vi "niRFUtil RFHS Channelizer ChannelizerArray CSG  phaseII.vi"(0 "Channelizer Ref":refnum<data-value>, 1 "Reset":bool, 2 "Benchmark Task":T2, 5 "Data":csg[](array[numeric]), 7 "Data Subset":T1={"Offset"=0, "Length"=-1}, 11 "error in (no error)":errorcluster, 13 "CPU Context":string) -> (4 "Channelizer Ref (out)":refnum<data-value>, 6 "Channel Data":csg[](array[numeric]), 8 "Channel Data Len":u32[](array[numeric]), 15 "error out":errorcluster)   [LabVIEW 2015, in "niRFUtil.lvlib"]
uses:
  niRFUtil.lvlib
  Utilities/Benchmark/niRFUtil RFHS Benchmark Task.ctl
  Utilities/niRFUtil RFHS Util Data Subset.ctl
  Includes/niRFUtil RFHS Channelizer ChannelizerInfo CSG.ctl
  Includes/niRFUtil RFHS Channelizer FilterRef.ctl
  Includes/niRFUtil RFHS Channelizer ChannelizerBufferingMode.ctl
  Utilities/Data FIFO/niRFUtil RFHS FIFO Reference.ctl
  Utilities/Data FIFO/niRFUtil RFHS FIFO.ctl
  Includes/niRFUtil RFHS Channelizer ChannelizerType.ctl
  Includes/niRFUtil RFHS Channelizer ChannelizerFlags.ctl
  niRFUtil RFHS Channelizer AdjustDataSubsetSpecification.vi
  niRFUtil RFHS Channelizer BufferLen CSG.vi
  niRFUtil RFHS Channelizer ChannelizerHandleDllError.vi
  Utilities/niRFUtil RFHS Util Process CPU Context.vi
  niRFUtil RFHS Channelizer ProcessCPUContext.vi
  Utilities/niRFUtil RFHS Util Dll Path.vi
panel:
  out "Time":u32
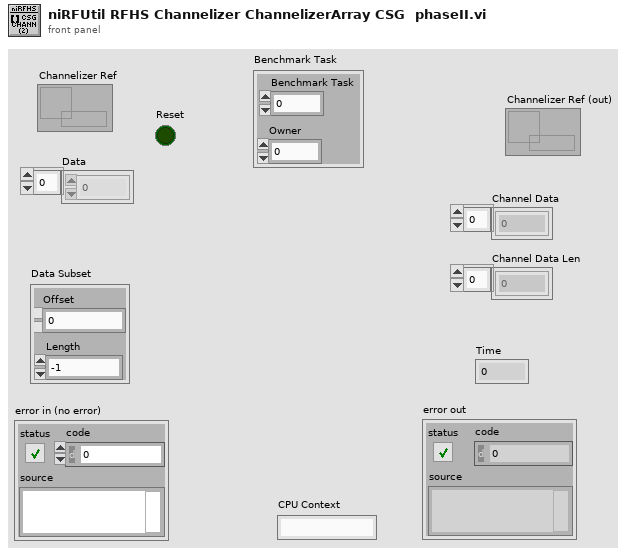
[diagram p1: front panel]
types:
  T1 = typedef "niRFUtil.lvlib/niRFUtil RFHS Util Data Subset.ctl" = cluster{"Offset":i32, "Length":i32}
  T2 = typedef "niRFUtil.lvlib/niRFUtil RFHS Benchmark Task.ctl" = cluster{"Benchmark Task":u64, "Owner":u32}
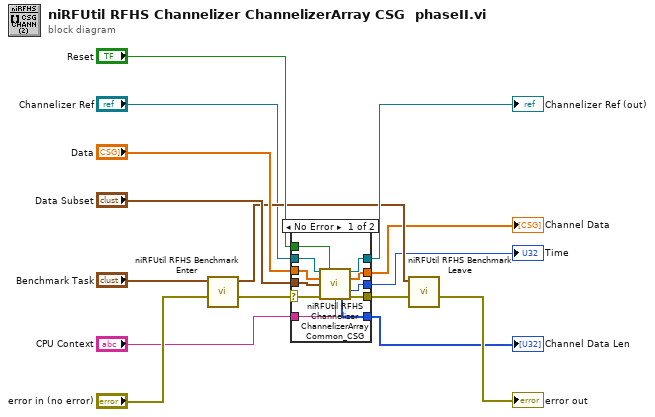
[diagram p0: block diagram]
diagram:
  n1 = call "niRFUtil RFHS Benchmark Enter.vi"("error in (no error)"="error in (no error)", "Benchmark Task (Parent)"="Benchmark Task") -> ("error out"=w1:errorcluster, "Benchmark Task (Self)"=w6:T2)  [unwired: 8 in]
  n2 = case shown="No Error" w1 {
    selector: w1 -> [w24 w28]
    tunnel: "Data" -> [w26 _]
    tunnel: "Reset" -> [w18 _]
    tunnel: [w23 w28] -> w12
    tunnel: "CPU Context" -> [w19 _]
    tunnel: "Data Subset" -> [w25 _]
    tunnel: "Channelizer Ref" -> [w16 w27]
    tunnel: [w22 w27] -> w7
    tunnel: [w21 _] -> w5
    tunnel: [w20 _] -> w4
    tunnel: [w17 _] -> w3
    frame No Error {
      n3 = call "niRFUtil RFHS Channelizer ChannelizerArrayCommon_CSG.vi"("Channelizer Ref"=w16, "Reset"=w18, "Data"=w26, "Data Subset"=w25, "error in (no error)"=w24, "CPU Context"=w19) -> ("Channelizer Ref (out)"=w22:refnum<data-value>, "Channel Data"=w21:csg[], "Time"=w20:u32, "Channel Data Len"=w17:u32[], "error out"=w23:errorcluster)  [unwired: 4 in, 1 out]
    }
    frame Error {
    }
  }
  "Channel Data" <- w5
  "Time" <- w4
  "Channelizer Ref (out)" <- w7
  "Channel Data Len" <- w3
  n4 = call "niRFUtil RFHS Benchmark Leave.vi"("error in (no error)"=w12, "Benchmark Task Self"=w6) -> ("error out"=→"error out":errorcluster)  [unwired: 8 in, 1 out]
